vi "Read Max.vi"(8 "error in (no error)":errorcluster, 11 "Tag in":refnum<class "Tag.lvclass">) -> (0 "error out":errorcluster, 2 "Max":variant, 3 "Tag out":refnum<class "Tag.lvclass">)   [LabVIEW 2018, in "Tag Engine.lvlib" / "Tag.lvclass"]
uses:
  Tag.lvclass
  Tag.lvclass/Tag.ctl
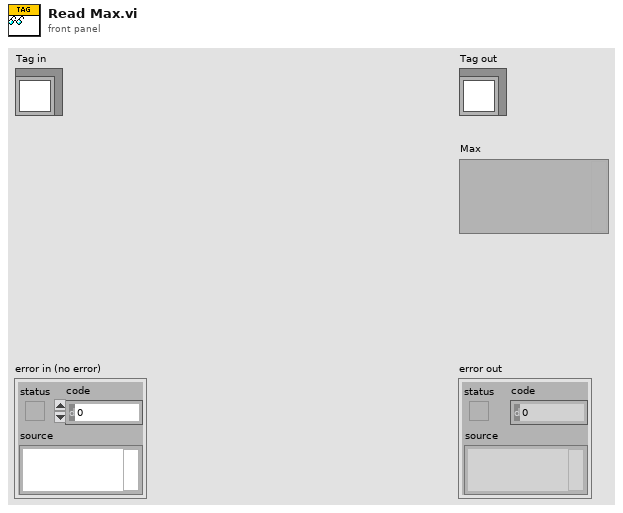
[diagram p1: front panel]
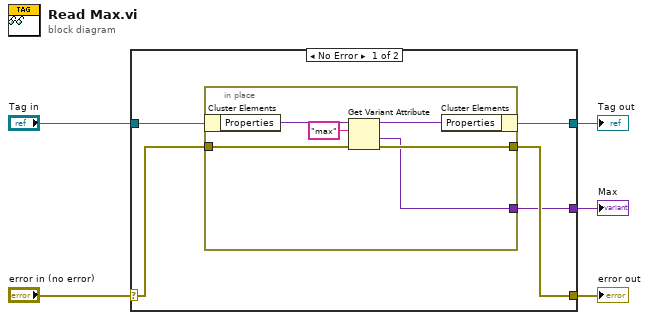
[diagram p0: block diagram]
diagram:
  n1 = case shown="No Error" "error in (no error)" {
    selector: "error in (no error)" -> [w8 w17]
    tunnel: [w7 w17] -> w4
    tunnel: [w9 w18] -> w2
    tunnel: "Tag in" -> [w10 w18]
    tunnel: [w6 _] -> w1
    frame No Error {
      n2 = in-place {
        in-place-border: w8 -> [w13]
        in-place-border: [w12] -> w7
        in-place-border: [w11] -> w6
        n3 = in-place-cluster #1(w10) -> ("Properties"=w16:variant)
        n4 = Get Variant Attribute(Variant=w16, name="max", error in=w13) -> (duplicate Variant=w14:variant, value=w11:variant, error out=w12:errorcluster)  [unwired: 1 in, 1 out]
        n5 = in-place-cluster #1("Properties"=w14) -> (w9:refnum<class "Tag.lvclass">)
      }
    }
    frame Error {
    }
  }
  "error out" <- w4
  "Tag out" <- w2
  "Max" <- w1
